vi "dfd_Util Cal CIC Output Params.vi"(8 "Output wl":i16, 11 "output MSB pos":i16) -> (0 "Shift":i16, 1 "length":i16, 2 "index":i16, 3 "zero padding":i16)   [LabVIEW 2017, in "NI_DigFilter_FXP.lvlib"]
uses:
  <vilib>/addons/Digital Filter Design/NI_DigFilter_FXP.lvlib
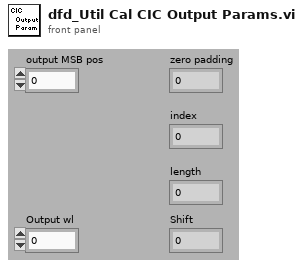
[diagram p1: front panel]
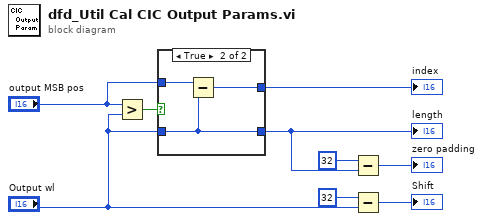
[diagram p0: block diagram]
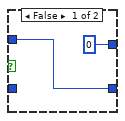
[diagram p2: hidden frame]
diagram:
  n1 = Greater?(x="output MSB pos", y="Output wl") -> (0:w2:bool)
  n2 = case shown="True" w2 {
    tunnel: "output MSB pos" -> [w10 w14]
    tunnel: "Output wl" -> [_ w12]
    tunnel: [i16 0 w13] -> w6
    tunnel: [w10 w12] -> w4
    frame False {
    }
    frame True {
      n3 = Subtract(x=w14, y=w12) -> (x-y=w13:i16)
    }
  }
  "index" <- w6
  "length" <- w4
  n4 = Subtract(x=i16 32, y=w4) -> (x-y=→"zero padding":i16)
  n5 = Subtract(x=i16 32, y="Output wl") -> (x-y=→"Shift":i16)
